vi "FixJKIHelper.vi"() -> ()   [LabVIEW 2014]
panel:
  out "size(s)":i32
  out "Numeric":i32
  out "Path":path
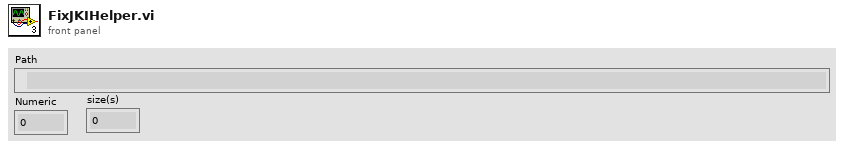
[diagram p1: front panel]
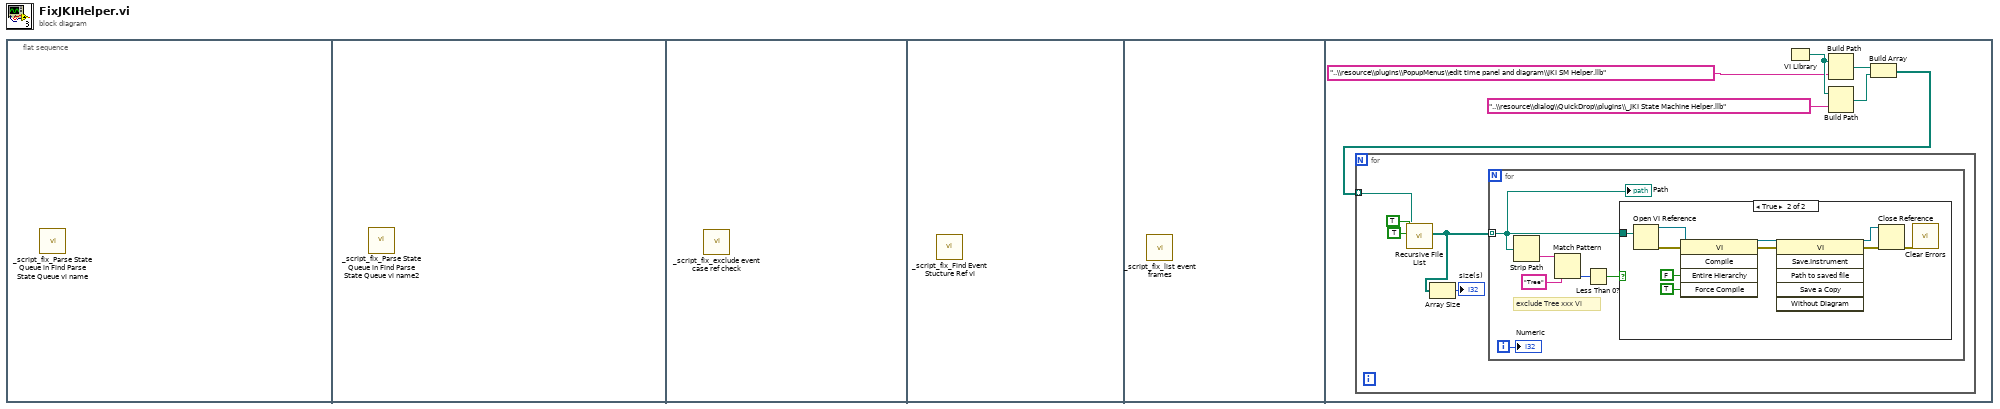
[diagram p0: block diagram]
diagram:
  n1 = flat-sequence {
    frame #0 {
      n2 = call "_script_fix_Parse State Queue in Find Parse State Queue vi name.vi"() -> ()  [unwired: 12 in]
    }
    frame #1 {
      n3 = call "_script_fix_Parse State Queue in Find Parse State Queue vi name2.vi"() -> ()  [unwired: 12 in]
    }
    frame #2 {
      n4 = call "_script_fix_exclude event case ref check.vi"() -> ()  [unwired: 12 in]
    }
    frame #3 {
      n5 = call "_script_fix_Find Event Stucture Ref vi.vi"() -> ()  [unwired: 12 in]
    }
    frame #4 {
      n6 = call "_script_fix_list event frames.vi"() -> ()  [unwired: 12 in]
    }
    frame #5 {
      n7 = VI Library() -> (path=w2:path)
      n8 = Build Path(base path=w2, name or relative path="..\\resource\\plugins\\PopupMenus\\edit time panel and diagram\\JKI SM Helper.llb") -> (appended path=w4:path)
      n9 = Build Path(base path=w2, name or relative path="..\\resource\\dialog\\QuickDrop\\plugins\\_JKI State Machine Helper.llb") -> (appended path=w6:path)
      n10 = Build Array(w4, w6) -> (w5:path[])
      n11 = for {
        tunnel: w5 -> [w9] mode=indexing
        n12 = call <vilib>:"Recursive File List.vi"("Continue Recursing on Error? (F)"=TRUE, "Treat LLBs as Folders?"=TRUE, "Folder Path"=w9) -> ("All Files in Dir"=w8:path[])  [unwired: 4 in, 4 out]
        n13 = Array Size(array=w8) -> (size(s)=→"size(s)":i32)
        n14 = for {
          tunnel: w8 -> [w16] mode=indexing
          i -> [w17]
          # "exclude Tree xxx Vi"
          n15 = Strip Path(path=w16) -> (name=w15:string)  [unwired: 1 out]
          n16 = Match Pattern(string=w15, regular expression="Tree") -> (offset past match=w13:i32)  [unwired: 1 in, 3 out]
          n17 = Less Than 0?(x=w13) -> (x < 0?=w12:bool)
          n18 = case shown="True" w12 {
            tunnel: w16 -> [_ w25]
            frame False {
            }
            frame True {
              n19 = Open VI Reference(vi path=w25) -> (vi reference=w23:refnum<vi>, error out=w24:errorcluster)  [unwired: 5 in]
              n20 = invoke class="VI" method="Compile"(reference=w23, error in=w24, "Entire Hierarchy"=FALSE ("Compile Entire Hierarchy (F)"), "Force Compile"=TRUE ("Force Compile (T)")) -> (reference out=w22:refnum<vi>, error out=w21:errorcluster)  [unwired: 1 in, 3 out]
              n21 = invoke class="VI" method="Save.Instrument"(reference=w22, error in=w21) -> (reference out=w19:refnum<vi>, error out=w20:errorcluster)  [unwired: 4 in, 4 out]
              n22 = Close Reference(reference=w19, error in (no error)=w20) -> (error out=w18:errorcluster)
              n23 = call <vilib>:"Clear Errors.vi"("error in (no error)"=w18) -> ()  [unwired: 5 in, 2 out]
            }
          }
          "Path" <- w16
          "Numeric" <- w17
        }
      }
    }
  }
